vi "LIA Debugging FPGA.vi"() -> ()   [LabVIEW 2018]
uses:
  <vilib>/eio/EIONode/EIONode.xnode
  <vilib>/rvi/eio/common/nirviEmuTemplateMethod_errors.vi
  <vilib>/Platform/TimedLoop/XDataNode/wakeup.ctl
  <vilib>/Platform/TimedLoop/XDataNode/XDNodeRunTimeDep.lvlib
  <vilib>/Platform/TimedLoop/XDataNode/nitl_modes.ctl
  <vilib>/Platform/TimedLoop/XDataNode/timing_clust.ctl
  <vilib>/Platform/TimedLoop/XDataNode/XDataNode.xnode
  <instrlib>/_niInstr/Basic Elements/v1/FPGA/niInstr Basic Elements v1 FPGA.lvlib
  <instrlib>/_niInstr/DSP/v1/Shared/Public/IQ Data.ctl
  <instrlib>/_niInstr/DSP/v1/Shared/niInstr DSP v1 Shared.lvlib
  <instrlib>/_niInstr/DSP/v1/FPGA/niInstr DSP v1 FPGA.lvlib
  <instrlib>/_niInstr/DSP/v1/Xnodes/Public/Frequency Shift/niInstr DSP v1 Frequency Shift FPGA.xnode
  Shared/_NI PLL IP/FPGA/NI PLL IP FPGA.lvlib
  <vilib>/rvi/FXPMathLib/FxpMul/XNode/nifxpmath_Multiplier.xnode
  <vilib>/rvi/FXPMathLib/FxpAdd/XNode/nifxpmath_Add.xnode
  <instrlib>/_niInstr/DSP/v1/FPGA/Public/Sub VIs/Frequency Shift/Frequency Shift - 2 spc.vi
  Shared/lib/fpga/Lock-In Amplifier Example FPGA.lvlib
  <instrlib>/_niInstr/Streaming/v1/Common/Stream State.ctl
  <instrlib>/_niInstr/Streaming/v1/Common/niInstr Streaming v1 Common.lvlib
  <vilib>/rvi/FXPMathLib/sim/FxpSim.dll
  <instrlib>/_niInstr/DSP/v1/FPGA/Public/Sub VIs/Fractional Decimator/Fractional Decimator - 10 cps - 1x oc.vi
  <instrlib>/_niInstr/DSP/v1/FPGA/Public/Sub VIs/Fractional Decimator/Fractional Decimator - 1 spc - 2x oc.vi
  <userlib>/_NI Noise Generation IP/FPGA/Public/Low Level/AWGN FXP23x2.vi
  <instrlib>/_niInstr/Data Trigger/v1/Shared/Public/Edge Configuration Trigger Slope.ctl
  <instrlib>/_niInstr/Data Trigger/v1/Shared/niInstr Data Trigger v1 Shared.lvlib
  <instrlib>/_niInstr/Data Trigger/v1/Shared/Public/Edge Configuration FXP(+-,18,1).ctl
  Shared/SOS/Controls/IIR_Coeffs.ctl
  LIA Decimator1 Enum.ctl
  LIA Decimator0 Enum.ctl
panel:
  out "stream.overflow? 0":bool
  in  "stream.clear overflow 0":bool
  in  "lock-in.iir enable0 0":bool
  in  "lock-in.iir enable1 0":bool
  in  "lock-in.iir config1 0":T1={"b0"=0.015777587890625, "b1"=-0.030517578125, "-a1"=1.9578399658203125, "-a2"=-0.9589080810546875}
  in  "lock-in.iir decimation1 0":fxp<+,4,4> format="%#_3g"
  in  "lock-in.iir decimation0 0":fxp<+,4,4> format="%#_3g"
  in  "lock-in.iir config0 0":T1={"b0"=0.015777587890625, "b1"=-0.030517578125, "-a1"=1.9578399658203125, "-a2"=-0.9589080810546875}
  in  "lock-in.decimator1 0":T2
  in  "lock-in.fir1 fs 0":fxp<+,48,1>
  in  "nco.enable 0":bool=TRUE
  in  "nco.reset 0":bool
  in  "nco.frequency 0":fxp<+/-,48,0>
  in  "lock-in.fir0 fs 0":fxp<+,48,1>
  in  "lock-in.decimator0 0":T3
  in  "dpll.reset 1":bool
  in  "dpll.enable 1":bool
  in  "dpll.q 1":fxp<+/-,48,0>
  in  "dpll.m 1":i8
  in  "dpll.config 1":T4
  out "dpll.vco output 1":fxp<+/-,48,0>
  in  "dpll.channel 1":i32
  in  "dpll.channel 0":i32
  out "dpll.vco output 0":fxp<+/-,48,0>
  in  "dpll.config 0":T4
  in  "dpll.m 0":i8
  in  "dpll.q 0":fxp<+/-,48,0>
  in  "dpll.enable 0":bool
  in  "dpll.reset 0":bool
  in  "lock-in.enable 3":bool
  in  "lock-in.enable 2":bool
  in  "lock-in.enable 1":bool
  in  "lock-in.carrier 3":fxp<+/-,48,0>
  in  "lock-in.carrier 2":fxp<+/-,48,0>
  in  "lock-in.enable 0":bool
  in  "lock-in.channel select 3":i32
  in  "lock-in.carrier select 3":i32
  in  "lock-in.cic config valid 3":bool
  in  "lock-in.cic config 3":cluster{"factor":fxp<+,16,16>, "shift":i16}
  in  "lock-in.reset 3":bool
  out "stream.state 3":T6 caption="stream.state 0"
  out "stream.samples transferred 3":u64 caption="stream.samples transferred 0"
  out "stream.metadata 3":u64 caption="stream.metadata 0"
  in  "stream.num samples 3":u64 caption="stream.num samples 0"
  in  "stream.request state 3":T6 caption="stream.request state 0"
  in  "lock-in.channel select 2":i32
  in  "lock-in.carrier select 2":i32
  in  "lock-in.cic config valid 2":bool
  in  "lock-in.cic config 2":cluster{"factor":fxp<+,16,16>, "shift":i16}
  in  "lock-in.reset 2":bool
  out "stream.state 2":T6 caption="stream.state 0"
  out "stream.samples transferred 2":u64 caption="stream.samples transferred 0"
  out "stream.metadata 2":u64 caption="stream.metadata 0"
  in  "stream.num samples 2":u64 caption="stream.num samples 0"
  in  "stream.request state 2":T6 caption="stream.request state 0"
  out "pll.vco output 0":fxp<+/-,48,0>
  out "pll.vco output 1":fxp<+/-,48,0>
  out "stream.metadata 4":u64 caption="stream.metadata 0"
  out "stream.samples transferred 4":u64 caption="stream.samples transferred 0"
  out "stream.state 4":T6 caption="stream.state 0"
  in  "stream.request state 4":T6 caption="stream.request state 0"
  in  "stream.num samples 4":u64 caption="stream.num samples 0"
  in  "preview.channel select":i32
  in  "ao.reset 3":bool
  in  "ao.carrier 2":fxp<+/-,48,0>=0.010000000000001563
  in  "ao.level 2":fxp<+/-,18,1>
  in  "ao.reset 2":bool
  in  "ao.carrier 1":fxp<+/-,48,0>=0.010000000000001563
  in  "ao.level 1":fxp<+/-,18,1>
  in  "ao.reset 1":bool
  in  "ao.reset 0":bool
  in  "ao.carrier 0":fxp<+/-,48,0>=0.010000000000001563
  in  "ao.level 0":fxp<+/-,18,1>
  in  "lock-in.channel select 1":i32
  in  "lock-in.channel select 0":i32
  in  "stream.request state 1":T6 caption="stream.request state 0"
  in  "stream.num samples 1":u64 caption="stream.num samples 0"
  out "stream.metadata 1":u64 caption="stream.metadata 0"
  out "stream.samples transferred 1":u64 caption="stream.samples transferred 0"
  out "stream.state 1":T6 caption="stream.state 0"
  in  "lock-in.reset 1":bool
  in  "lock-in.cic config 1":cluster{"factor":fxp<+,16,16>, "shift":i16}
  in  "lock-in.cic config valid 1":bool
  in  "lock-in.carrier select 1":i32
  in  "lock-in.carrier select 0":i32
  in  "lock-in.cic config valid 0":bool
  in  "lock-in.cic config 0":cluster{"factor":fxp<+,16,16>, "shift":i16}
  in  "lock-in.reset 0":bool
  in  "lock-in.carrier 1":fxp<+/-,48,0>
  in  "lock-in.carrier 0":fxp<+/-,48,0>
  in  "ao.level 3":fxp<+/-,18,1>
  in  "pll.channel 1":i32
  in  "pll.reset 1":bool
  in  "pll.enable 1":bool
  in  "pll.config 1":T7={"quiescent frequency"=0.10000000000000142, "compensation"=0.0, "psd gain"=-18, "loop filter"={"order"=4, "cutoff"=6}}
  in  "pll.channel 0":i32
  in  "ao.noise gain 3":fxp<+,18,1>=0.01000213623046875
  in  "ao.carrier 3":fxp<+/-,48,0>=0.010000000000001563
  in  "ao.noise seeds 3":fxp<+,23,23>[](array[numeric])=[1.0, 12323.0]
  in  "pll.reset 0":bool
  in  "pll.enable 0":bool
  in  "stream.request state 0":T6
  in  "stream.num samples 0":u64
  out "stream.metadata 0":u64
  out "stream.samples transferred 0":u64
  out "stream.state 0":T6
  in  "pll.config 0":T7={"quiescent frequency"=0.10000000000000142, "compensation"=0.0, "psd gain"=-18, "loop filter"={"order"=4, "cutoff"=6}}
  out "IO Module\\InitDone":bool
  out "IO Module\\User Error":u32
  in  "IO Module\\User Command":u32
  in  "IO Module\\User Command Valid":bool
  out "IO Module\\User Command Ready":bool
  in  "IO Module\\User Command Arg 0":u32
  in  "IO Module\\User Command Arg 1":u32
  out "IO Module\\User Command Error":u16
  out "IO Module\\User Command Return":u32
  out "IO Module\\User Command Return Valid":bool
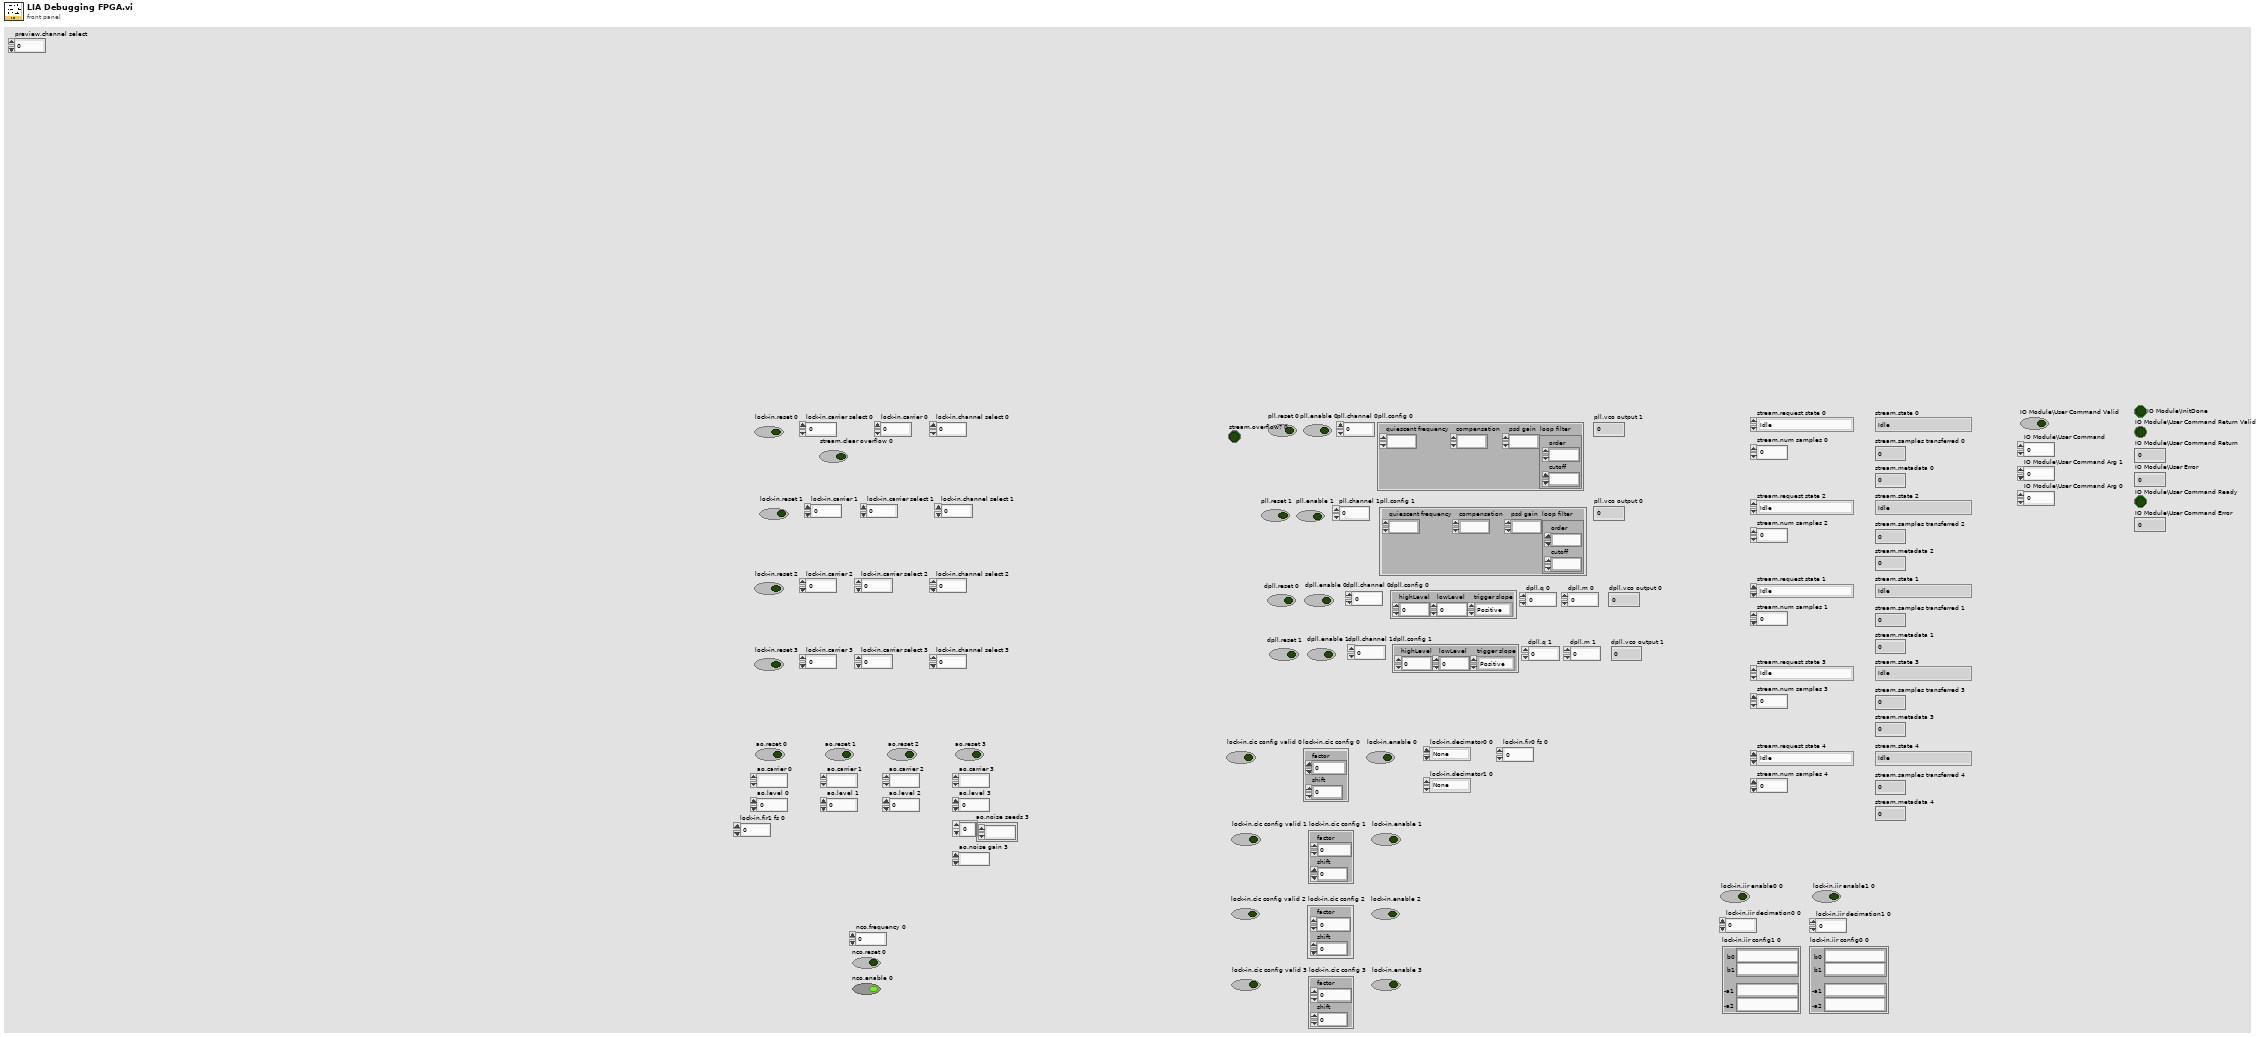
[diagram p1: front panel]
types:
  T1 = typedef "IIR_Coeffs.ctl" = cluster{"b0":fxp<+/-,18,2>, "b1":fxp<+/-,18,2>, "-a1":fxp<+/-,18,2>, "-a2":fxp<+/-,18,2>}
  T2 = typedef "LIA Decimator1 Enum.ctl" = enum16{"None", "FIR", "SOS"}
  T3 = typedef "LIA Decimator0 Enum.ctl" = enum16{"None", "CIC", "FIR", "4HB", "SOS", "4SOS"}
  T4 = typedef "niInstr Data Trigger v1 Shared.lvlib/Edge Configuration FXP(+-,18,1).ctl" = cluster{"highLevel":fxp<+/-,18,1>, "lowLevel":fxp<+/-,18,1>, "trigger slope":T5}
  T5 = typedef "niInstr Data Trigger v1 Shared.lvlib/Edge Configuration Trigger Slope.ctl" = enum8{"Positive", "Negative"}
  T6 = typedef "niInstr Streaming v1 Common.lvlib/Stream State.ctl" = enum8{"Idle", "Finite Transfer", "Continuous", "Done", "Error", "Not Ready", "Cancel"}
  T7 = cluster{"quiescent frequency":fxp<+/-,48,0>, "compensation":fxp<+/-,18,3>, "psd gain":i16, "loop filter":cluster{"order":i32, "cutoff":i8}}
  T8 = typedef "XDNodeRunTimeDep.lvlib/timing_clust.ctl" = cluster{"Expected End [f-1]":u64, "Actual End [f-1]":u64, "Finished Late? [f-1]":bool, "Expected End [i-1]":u64, "Actual End [i-1]":u64, "Finished Late? [i-1]":bool, "Expected Start [i]":u64, "Actual Start [i]":u64, "Expected Start [f]":u64, "Actual Start [f]":u64, "Source Name":string, "Structure Name":string, "Period":i64, "Deadline":i64, "Offset":i64, "Start":i64, "Priority":i32, "Timeout":i32, "Mode":T9, "Wakeup Reason":T10, "Error":errorcluster, "Source Type":string, "Secondary Source Type":string, "Global End Time":u64, "Global Start Time":u64, "Frame Duration":u64, "Iteration Duration":u64, "Assigned CPU":i32, "I/O Scan Engine Mode":u32}
  T9 = typedef "XDNodeRunTimeDep.lvlib/nitl_modes.ctl" = enum32{"No Change", "Process missed periods, maintain original phase", "Discard missed periods, maintain original phase", "Process missed periods, ignore original phase", "Discard missed periods, ignore original phase"}
  T10 = typedef "XDNodeRunTimeDep.lvlib/wakeup.ctl" = enum32{"Normal", "Aborted", "Asynchronous wakeup", "Timing source error", "Timed loop error", "Timeout"}
  T11 = cluster{"stream.num samples 0":u64, "stream.request state 0":T6, "stream.index 0":i16}
  T12 = typedef "niInstr DSP v1 Shared.lvlib/IQ Data.ctl" = cluster{"I":fxp<+/-,18,1>, "Q":fxp<+/-,18,1>, "overflow":bool}
  T13 = cluster{"stream.metadata 0":u64, "stream.samples transferred 0":u64, "stream.state 0":T6}
  T14 = typedef "niInstr DSP v1 Shared.lvlib/IQ Data - 25 bit.ctl" = cluster{"I":fxp<+/-,25,1>, "Q":fxp<+/-,25,1>, "overflow":bool}
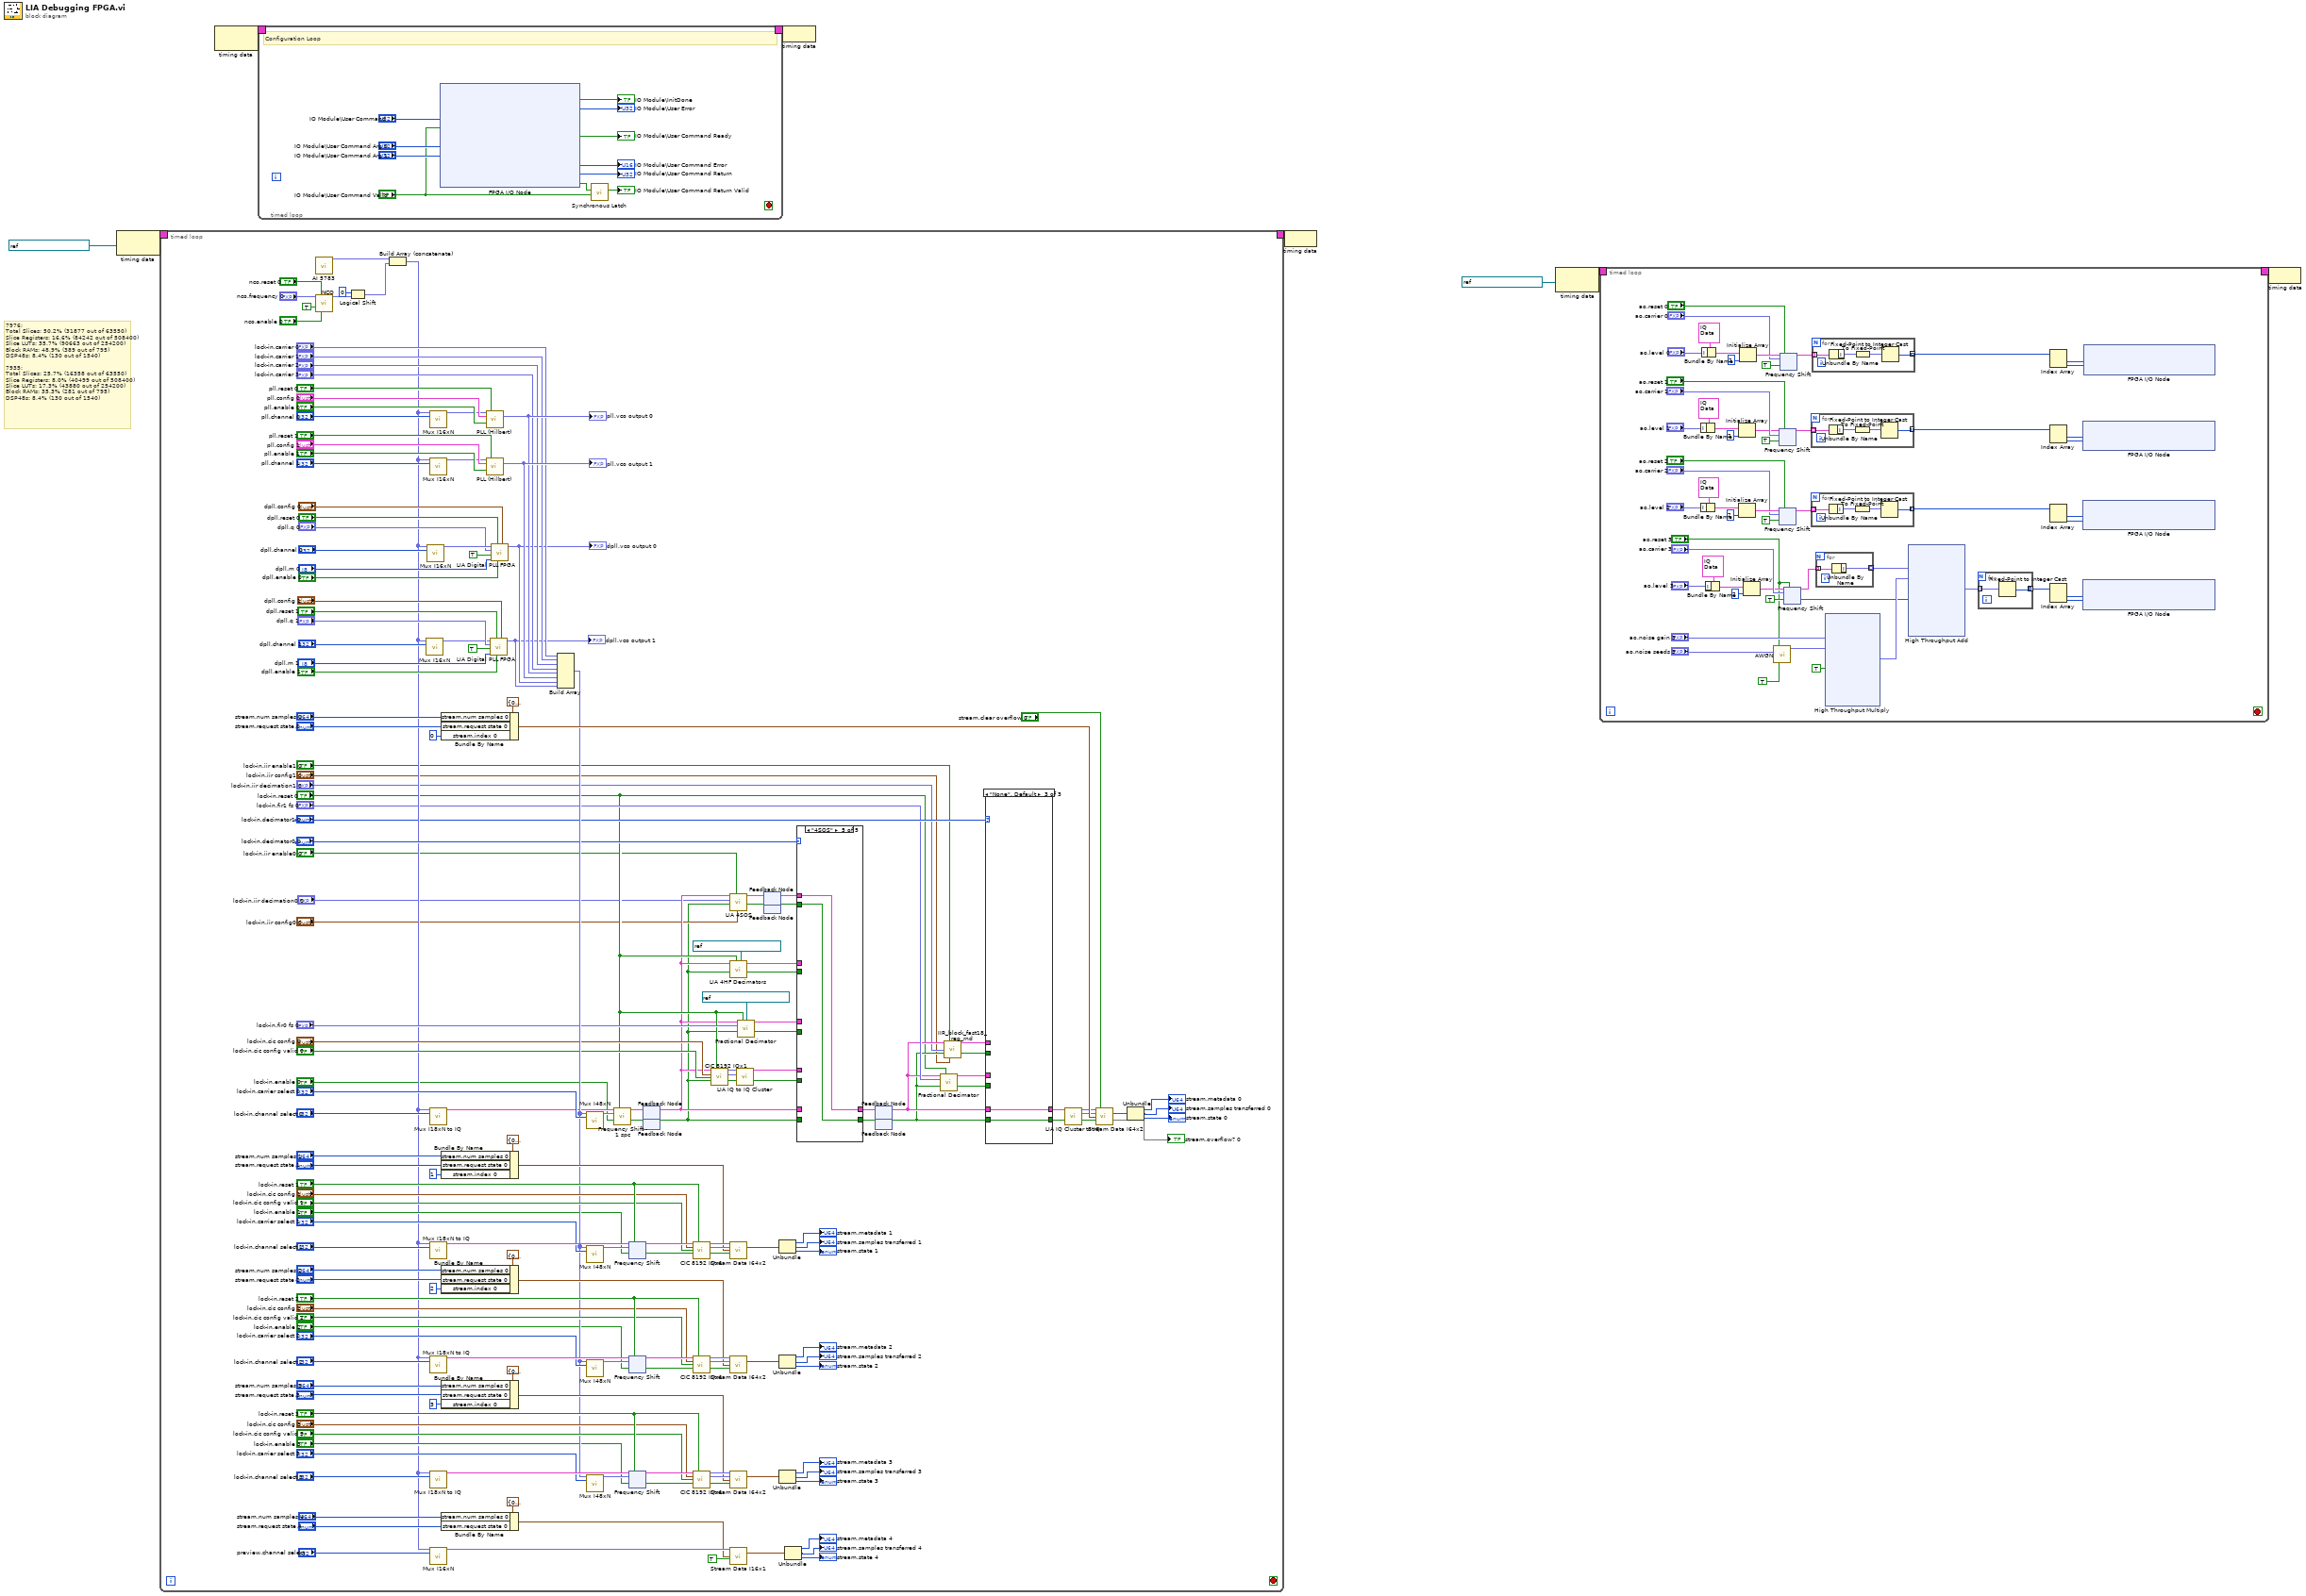
[diagram p0: block diagram]
diagram:
  # "7976:\nTotal Slices: 50.2% (31877 out of 63550)\nSlice Registers: 16.6% (84242 out of 508400)\nSlice LUTs: 35.7% (90663 out of 254200)\nBlock RAMs: 48.9% (389 out of 795)\nDSP48s: 8.4% (130 out of 1540)\n\n7935:\nTotal Slices: 25.7% (16358 out of 63550)\nSlice Registers: 8.0% (40499 out of 508400)\nSlice LUTs: 17.3% (43880 out of 254200)\nBlock RAMs: 35.3% (281 out of 795)\nDSP48s: 8.4% (130 out of 1540)"
  n1 = node-c288(refnum<k21> "IO Module\\Data Clock" ("Source Name")) -> (w8:T8)
  n2 = timed-loop {
    timing: w8 -> [_]
    timing-out: [_] -> w7
    stop <- _ stop-if-true
    n3 = call "AI 5783.vi"() -> ("i18x1"=w66:fxp<+/-,18,1>[])  [unwired: 14 in, 1 out]
    n4 = call <instrlib>:"NCO.vi"("frequency"="nco.frequency 0", "reset"="nco.reset 0", "input valid"=TRUE, "enable (T)"="nco.enable 0") -> ("cosine out"=w39:fxp<+/-,18,1>)  [unwired: 9 in, 2 out]
    n5 = Logical Shift(y=i16 0, x=w39) -> (x << y=w40:fxp<+/-,18,1>)
    n6 = Build Array (concatenate)(w66, w40) -> (w59:fxp<+/-,18,1>[])
    n7 = call "Mux I16xN.vi"("i16xn in"=w59, "index"="dpll.channel 1") -> ("i16 out"=w69:fxp<+/-,18,1>)  [unwired: 12 in, 1 out]
    n8 = call "Mux I16xN.vi"("i16xn in"=w59, "index"="dpll.channel 0") -> ("i16 out"=w81:fxp<+/-,18,1>)  [unwired: 12 in, 1 out]
    n9 = call "Mux I16xN.vi"("i16xn in"=w59, "index"="pll.channel 0") -> ("i16 out"=w185:fxp<+/-,18,1>)  [unwired: 12 in, 1 out]
    n10 = call "Mux I16xN.vi"("i16xn in"=w59, "index"="pll.channel 1") -> ("i16 out"=w179:fxp<+/-,18,1>)  [unwired: 12 in, 1 out]
    n11 = call "Mux I18xN to IQ.vi"("i16xn in"=w59, "index"="lock-in.channel select 0") -> ("output"=w28:T12)  [unwired: 12 in, 1 out]
    n12 = call "Mux I18xN to IQ.vi"("i16xn in"=w59, "index"="lock-in.channel select 1") -> ("output"=w167:T12)  [unwired: 12 in, 1 out]
    n13 = call "Mux I18xN to IQ.vi"("i16xn in"=w59, "index"="lock-in.channel select 2") -> ("output"=w133:T12)  [unwired: 12 in, 1 out]
    n14 = call "Mux I18xN to IQ.vi"("i16xn in"=w59, "index"="lock-in.channel select 3") -> ("output"=w112:T12)  [unwired: 12 in, 1 out]
    n15 = call "Mux I16xN.vi"("i16xn in"=w59, "index"="preview.channel select") -> ("i16 out"=w141:fxp<+/-,18,1>)  [unwired: 12 in, 1 out]
    n16 = Bundle By Name(cluster=T11 {"stream.num samples 0"=0, "stream.request state 0"=enum."Idle", "stream.index 0"=0} ("config"), "stream.num samples 0"="stream.num samples 0", "stream.request state 0"="stream.request state 0", "stream.index 0"=i16 0) -> (w170:T11)
    n17 = Bundle By Name(cluster=T11 {"stream.num samples 0"=0, "stream.request state 0"=enum."Idle", "stream.index 0"=0} ("config"), "stream.num samples 0"="stream.num samples 1", "stream.request state 0"="stream.request state 1", "stream.index 0"=i16 1) -> (w149:T11)
    n18 = Bundle By Name(cluster=T11 {"stream.num samples 0"=0, "stream.request state 0"=enum."Idle", "stream.index 0"=0} ("config"), "stream.num samples 0"="stream.num samples 2", "stream.request state 0"="stream.request state 2", "stream.index 0"=i16 2) -> (w115:T11)
    n19 = Bundle By Name(cluster=T11 {"stream.num samples 0"=0, "stream.request state 0"=enum."Idle", "stream.index 0"=0} ("config"), "stream.num samples 0"="stream.num samples 3", "stream.request state 0"="stream.request state 3", "stream.index 0"=i16 3) -> (w94:T11)
    n20 = Bundle By Name(cluster=T11 {"stream.num samples 0"=0, "stream.request state 0"=enum."Idle", "stream.index 0"=0} ("config"), "stream.num samples 0"="stream.num samples 4", "stream.request state 0"="stream.request state 4") -> (w137:T11)
    n21 = call "PLL (Hilbert).vi"("input"=w185, "reset"="pll.reset 0", "config"="pll.config 0", "enable"="pll.enable 0") -> ("output"=w134:fxp<+/-,48,0>)  [unwired: 11 in]
    "pll.vco output 0" <- w134
    n22 = call "PLL (Hilbert).vi"("input"=w179, "reset"="pll.reset 1", "config"="pll.config 1", "enable"="pll.enable 1") -> ("output"=w135:fxp<+/-,48,0>)  [unwired: 11 in]
    "pll.vco output 1" <- w135
    n23 = call "LIA Digital PLL FPGA.vi"("configuration"="dpll.config 1", "arm"="dpll.enable 1", "reset"="dpll.reset 1", "m"="dpll.m 1", "input valid"=TRUE, "q"="dpll.q 1", "I"=w69) -> ("frequency shift"=w65:fxp<+/-,48,0>)  [unwired: 1 in, 3 out]
    "dpll.vco output 1" <- w65
    n24 = call "LIA Digital PLL FPGA.vi"("configuration"="dpll.config 0", "arm"="dpll.enable 0", "reset"="dpll.reset 0", "m"="dpll.m 0", "input valid"=TRUE, "q"="dpll.q 0", "I"=w81) -> ("frequency shift"=w76:fxp<+/-,48,0>)  [unwired: 1 in, 3 out]
    "dpll.vco output 0" <- w76
    n25 = Build Array("lock-in.carrier 0", "lock-in.carrier 1", "lock-in.carrier 2", "lock-in.carrier 3", w134, w135, w76, w65) -> (w91:fxp<+/-,48,0>[])
    n26 = call "Mux I48xN.vi"("i48xn in"=w91, "index"="lock-in.carrier select 0") -> ("i48 out"=w25:fxp<+/-,48,0>)  [unwired: 13 in]
    n27 = call "Mux I48xN.vi"("i48xn in"=w91, "index"="lock-in.carrier select 1") -> ("i48 out"=w166:fxp<+/-,48,0>)  [unwired: 13 in]
    n28 = call "Mux I48xN.vi"("i48xn in"=w91, "index"="lock-in.carrier select 2") -> ("i48 out"=w132:fxp<+/-,48,0>)  [unwired: 13 in]
    n29 = call "Mux I48xN.vi"("i48xn in"=w91, "index"="lock-in.carrier select 3") -> ("i48 out"=w111:fxp<+/-,48,0>)  [unwired: 13 in]
    n30 = call <instrlib>:"Frequency Shift - 1 spc.vi"("data in"=w28, "reset"="lock-in.reset 0", "frequency shift"=w25, "input valid"="lock-in.enable 0") -> ("data out"=w27:T12, "output valid"=w26:bool)  [unwired: 8 in, 2 out]
    n31 = xnode "Frequency Shift"("data in"=w167, "reset"="lock-in.reset 1", "frequency shift"=w166, "input valid"="lock-in.enable 1") -> ("data out"=w165:T12, "output valid"=w164:bool)  [unwired: 2 in, 1 out]
    n32 = xnode "Frequency Shift"("data in"=w133, "reset"="lock-in.reset 2", "frequency shift"=w132, "input valid"="lock-in.enable 2") -> ("data out"=w131:T12, "output valid"=w130:bool)  [unwired: 2 in, 1 out]
    n33 = xnode "Frequency Shift"("data in"=w112, "reset"="lock-in.reset 3", "frequency shift"=w111, "input valid"="lock-in.enable 3") -> ("data out"=w110:T12, "output valid"=w109:bool)  [unwired: 2 in, 1 out]
    n34 = feedback-in #1(w27) -> ()
    n35 = feedback #1() -> (w17:T12)  [unwired: 1 in]
    n36 = feedback-in #2(w26) -> ()
    n37 = feedback #2() -> (w12:bool)  [unwired: 1 in]
    n38 = call "CIC 8192 IQx1.vi"("data"=w165, "reset"="lock-in.reset 1", "config"="lock-in.cic config 1", "config valid"="lock-in.cic config valid 1", "input valid"=w164) -> ("i out"=w160:fxp<+/-,64,1>, "q out"=w159:fxp<+/-,64,1>, "output valid"=w158:bool)  [unwired: 8 in]
    n39 = call "CIC 8192 IQx1.vi"("data"=w131, "reset"="lock-in.reset 2", "config"="lock-in.cic config 2", "config valid"="lock-in.cic config valid 2", "input valid"=w130) -> ("i out"=w126:fxp<+/-,64,1>, "q out"=w125:fxp<+/-,64,1>, "output valid"=w124:bool)  [unwired: 8 in]
    n40 = call "CIC 8192 IQx1.vi"("data"=w110, "reset"="lock-in.reset 3", "config"="lock-in.cic config 3", "config valid"="lock-in.cic config valid 3", "input valid"=w109) -> ("i out"=w105:fxp<+/-,64,1>, "q out"=w104:fxp<+/-,64,1>, "output valid"=w103:bool)  [unwired: 8 in]
    n41 = call "CIC 8192 IQx1.vi"("data"=w17, "reset"="lock-in.reset 0", "config"="lock-in.cic config 0", "config valid"="lock-in.cic config valid 0", "input valid"=w12) -> ("i out"=w46:fxp<+/-,64,1>, "q out"=w45:fxp<+/-,64,1>, "output valid"=w61:bool)  [unwired: 8 in]
    n42 = call "LIA 4HF Decimators.vi"("clock x 2"=refnum<k21> "IO Module\\Data Clock 2x", "reset"="lock-in.reset 0", "input valid"=w12, "data in"=w17) -> ("output valid"=w50:bool, "data out"=w51:T12)  [unwired: 6 in]
    n43 = call "LIA 4SOS.vi"("lock-in.iir config0 0"="lock-in.iir config0 0", "lock-in.iir enable0 0"="lock-in.iir enable0 0", "input valid"=w12, "lock-in.iir decimation0 0"="lock-in.iir decimation0 0", "IQ_Data_In"=w17) -> ("output valid"=w14:bool, "IQ_Data_Out"=w15:T12)  [unwired: 5 in]
    n44 = call "Stream Data I64x2.vi"("i in"=w160, "q in"=w159, "config"=w149, "input valid"=w158) -> ("status"=w157:T13)  [unwired: 11 in]
    n45 = call "Stream Data I64x2.vi"("i in"=w126, "q in"=w125, "config"=w115, "input valid"=w124) -> ("status"=w123:T13)  [unwired: 11 in]
    n46 = call "Stream Data I64x2.vi"("i in"=w105, "q in"=w104, "config"=w94, "input valid"=w103) -> ("status"=w102:T13)  [unwired: 11 in]
    n47 = call "Stream Data I16x1.vi"("i in"=w141, "config"=w137, "input valid"=TRUE) -> ("status"=w143:T13)  [unwired: 12 in]
    n48 = call "LIA IQ to IQ Cluster.vi"("i in"=w46, "q in"=w45) -> ("data out"=w44:T12)  [unwired: 13 in]
    n49 = call-poly <instrlib>:"Fractional Decimator.vi"("data in"=w17, "reset"="lock-in.reset 0", "clock x 2"=refnum<k21> "IO Module\\Data Clock 2x", "output sample rate"="lock-in.fir0 fs 0", "input valid"=w12) -> ("data out"=w53:T12, "output valid"=w54:bool)  [unwired: 8 in, 1 out]
    n50 = feedback-in #3(w15) -> ()
    n51 = feedback #3() -> (w10:T12)  [unwired: 1 in]
    n52 = feedback-in #4(w14) -> ()
    n53 = feedback #4() -> (w9:bool)  [unwired: 1 in]
    n54 = Unbundle(w157) -> ("stream.metadata 0"=→"stream.metadata 1":u64, "stream.samples transferred 0"=→"stream.samples transferred 1":u64, "stream.state 0"=→"stream.state 1":T6)
    n55 = Unbundle(w123) -> ("stream.metadata 0"=→"stream.metadata 2":u64, "stream.samples transferred 0"=→"stream.samples transferred 2":u64, "stream.state 0"=→"stream.state 2":T6)
    n56 = Unbundle(w102) -> ("stream.metadata 0"=→"stream.metadata 3":u64, "stream.samples transferred 0"=→"stream.samples transferred 3":u64, "stream.state 0"=→"stream.state 3":T6)
    n57 = Unbundle(w143) -> ("stream.metadata 0"=→"stream.metadata 4":u64, "stream.samples transferred 0"=→"stream.samples transferred 4":u64, "stream.state 0"=→"stream.state 4":T6)
    n58 = case shown="\"4SOS\"" "lock-in.decimator0 0" {
      tunnel: [w196 w198 w200 w202 w203] -> w33
      tunnel: w61 -> [_ w198 _ _ _]
      tunnel: w54 -> [_ _ w200 _ _]
      tunnel: w12 -> [w196 _ _ _ _]
      tunnel: w53 -> [_ _ w199 _ _]
      tunnel: w17 -> [w195 _ _ _ _]
      tunnel: w51 -> [_ _ _ w201 _]
      tunnel: w50 -> [_ _ _ w202 _]
      tunnel: [w195 w197 w199 w201 w204] -> w35
      tunnel: w44 -> [_ w197 _ _ _]
      tunnel: w10 -> [_ _ _ _ w204]
      tunnel: w9 -> [_ _ _ _ w203]
      frame "None", Default {
      }
      frame "CIC" {
      }
      frame "FIR" {
      }
      frame "4HB" {
      }
      frame "4SOS" {
      }
    }
    n59 = feedback #5() -> (w34:T12)  [unwired: 1 in]
    n60 = feedback-in #5(w35) -> ()
    n61 = feedback #6() -> (w32:bool)  [unwired: 1 in]
    n62 = feedback-in #6(w33) -> ()
    n63 = call-poly <instrlib>:"Fractional Decimator.vi"("data in"=w34, "reset"="lock-in.reset 0", "output sample rate"="lock-in.fir1 fs 0", "input valid"=w32) -> ("data out"=w43:T14, "output valid"=w42:bool)  [unwired: 9 in, 1 out]
    n64 = call "IIR_block_fast18_reg_rnd.vi"("IQ_Data_In"=w34, "enable"="lock-in.iir enable1 0", "Decimation Factor (-1)"="lock-in.iir decimation1 0", "Valid In"=w32, "IIR 2 coeffs"="lock-in.iir config1 0") -> ("IQ_Data_Out"=w37:T12, "output valid"=w36:bool)  [unwired: 9 in]
    n65 = case shown="\"None\", Default" "lock-in.decimator1 0" {
      tunnel: [w189 w191 w194] -> w49
      tunnel: w32 -> [_ _ w194]
      tunnel: w34 -> [_ _ w193]
      tunnel: [w190 w192 w193] -> w22
      tunnel: w43 -> [w190 _ _]
      tunnel: w42 -> [w189 _ _]
      tunnel: w37 -> [_ w192 _]
      tunnel: w36 -> [_ w191 _]
      frame "FIR" {
      }
      frame "SOS" {
      }
      frame "None", Default {
      }
    }
    n66 = call "LIA IQ Cluster to IQ.vi"("data in"=w22) -> ("i in"=w21:fxp<+/-,64,1>, "q in"=w20:fxp<+/-,64,1>)  [unwired: 13 in]
    n67 = call "Stream Data I64x2.vi"("i in"=w21, 1:"stream.clear overflow 0", "q in"=w20, "config"=w170, "input valid"=w49) -> ("status"=w178:T13, 10:→"stream.overflow? 0")  [unwired: 9 in]
    n68 = Unbundle(w178) -> ("stream.metadata 0"=→"stream.metadata 0":u64, "stream.samples transferred 0"=→"stream.samples transferred 0":u64, "stream.state 0"=→"stream.state 0":T6)
  }
  n69 = node-c288() -> (w2:T8)  [unwired: 1 in]
  n70 = timed-loop {
    timing: w2 -> [_]
    timing-out: [_] -> w1
    stop <- _ stop-if-true
    # "Configuration Loop"
    n71 = xnode "FPGA I/O Node"("IO Module\\User Command"="IO Module\\User Command", "IO Module\\User Command Valid"="IO Module\\User Command Valid", "IO Module\\User Command Arg 0"="IO Module\\User Command Arg 0", "IO Module\\User Command Arg 1"="IO Module\\User Command Arg 1") -> ("IO Module\\InitDone"=→"IO Module\\InitDone":bool, "IO Module\\Clip Error Code"=→"IO Module\\User Error":u32, "IO Module\\User Command Ready"=→"IO Module\\User Command Ready":bool, "IO Module\\User Command Error"=→"IO Module\\User Command Error":u16, "IO Module\\User Command Return"=→"IO Module\\User Command Return":u32, "IO Module\\User Command Return Valid"=w235:bool)  [unwired: 10 in, 10 out]
    n72 = call <instrlib>:"Synchronous Latch.vi"("clear"="IO Module\\User Command Valid", "set"=w235) -> ("out"=→"IO Module\\User Command Return Valid":bool)  [unwired: 9 in]
  }
  n73 = node-c288(w1) -> ()
  n74 = node-c288(w7) -> ()
  n75 = node-c288(refnum<k21> "IO Module\\Data Clock" ("Source Name")) -> (w5:T8)
  n76 = timed-loop {
    timing: w5 -> [_]
    timing-out: [_] -> w4
    stop <- _ stop-if-true
    n77 = Bundle By Name(cluster=T12 {"I"=0.0, "Q"=0.0, "overflow"=FALSE} ("output"), "I"="ao.level 1") -> (w268:T12)
    n78 = Bundle By Name(cluster=T12 {"I"=0.0, "Q"=0.0, "overflow"=FALSE} ("output"), "I"="ao.level 2") -> (w258:T12)
    n79 = Bundle By Name(cluster=T12 {"I"=0.0, "Q"=0.0, "overflow"=FALSE} ("output"), "I"="ao.level 0") -> (w283:T12)
    n80 = Bundle By Name(cluster=T12 {"I"=0.0, "Q"=0.0, "overflow"=FALSE} ("output"), "I"="ao.level 3") -> (w292:T12)
    n81 = Initialize Array(w268, 2 ("dimension size")) -> (w264:T12[])
    n82 = Initialize Array(w258, 2 ("dimension size")) -> (w262:T12[])
    n83 = Initialize Array(w283, 2 ("dimension size")) -> (w287:T12[])
    n84 = Initialize Array(w292, 2 ("dimension size")) -> (w288:T12[])
    n85 = call-poly <userlib>:"AWGN.vi"("reset"="ao.reset 3", "seeds"="ao.noise seeds 3", "ready"=TRUE) -> ("output 0"=w295:fxp<+/-,23,4>[])  [unwired: 10 in, 2 out]
    n86 = xnode "Frequency Shift"("data in"=w264, "reset"="ao.reset 1", "frequency shift"="ao.carrier 1", "input valid"=TRUE) -> ("data out"=w272:T12[])  [unwired: 2 in, 2 out]
    n87 = xnode "Frequency Shift"("data in"=w262, "reset"="ao.reset 2", "frequency shift"="ao.carrier 2", "input valid"=TRUE) -> ("data out"=w254:T12[])  [unwired: 2 in, 2 out]
    n88 = xnode "Frequency Shift"("data in"=w287, "reset"="ao.reset 0", "frequency shift"="ao.carrier 0", "input valid"=TRUE) -> ("data out"=w279:T12[])  [unwired: 2 in, 2 out]
    n89 = xnode "Frequency Shift"("data in"=w288, "reset"="ao.reset 3", "frequency shift"="ao.carrier 3", "input valid"=TRUE) -> ("data out"=w303:T12[], "output valid"=w300:bool)  [unwired: 2 in, 1 out]
    n90 = for {
      tunnel: w272 -> [w319] mode=indexing
      tunnel: [w320] -> w273 mode=indexing
      n91 = Unbundle By Name(w319) -> ("I"=w318:fxp<+/-,18,1>)
      n92 = To Fixed-Point(number=w318) -> (fixed-point=w317:fxp<+/-,16,1>)  [unwired: 1 in]
      n93 = Fixed-Point to Integer Cast(1:w317) -> (0:w320:i16)
    }
    n94 = for {
      tunnel: w254 -> [w306] mode=indexing
      tunnel: [w307] -> w253 mode=indexing
      n95 = Unbundle By Name(w306) -> ("I"=w305:fxp<+/-,18,1>)
      n96 = To Fixed-Point(number=w305) -> (fixed-point=w304:fxp<+/-,16,1>)  [unwired: 1 in]
      n97 = Fixed-Point to Integer Cast(1:w304) -> (0:w307:i16)
    }
    n98 = for {
      tunnel: w279 -> [w332] mode=indexing
      tunnel: [w333] -> w278 mode=indexing
      n99 = Unbundle By Name(w332) -> ("I"=w331:fxp<+/-,18,1>)
      n100 = To Fixed-Point(number=w331) -> (fixed-point=w330:fxp<+/-,16,1>)  [unwired: 1 in]
      n101 = Fixed-Point to Integer Cast(1:w330) -> (0:w333:i16)
    }
    n102 = for {
      tunnel: w303 -> [w346] mode=indexing
      tunnel: [w345] -> w299 mode=indexing
      n103 = Unbundle By Name(w346) -> ("I"=w345:fxp<+/-,18,1>)
    }
    n104 = xnode ("High Throughput Multiply")("x"="ao.noise gain 3", "y"=w295, "input valid"=TRUE) -> ("x*y"=w302:fxp<+/-,41,5>[])  [unwired: 1 in, 2 out]
    n105 = xnode ("High Throughput Add")("x"=w299, "y"=w302, "input valid"=w300) -> ("x+y"=w294:fxp<+/-,16,1>[])  [unwired: 1 in, 2 out]
    n106 = for {
      tunnel: w294 -> [w344] mode=indexing
      tunnel: [w343] -> w263 mode=indexing
      n107 = Fixed-Point to Integer Cast(1:w344) -> (0:w343:i16)
    }
    n108 = Index Array(array=w278) -> (element #1=w277:i16, element #2=w276:i16)  [unwired: 2 in]
    n109 = Index Array(array=w273) -> (element #1=w274:i16, element #2=w275:i16)  [unwired: 2 in]
    n110 = Index Array(array=w253) -> (element #1=w252:i16, element #2=w251:i16)  [unwired: 2 in]
    n111 = Index Array(array=w263) -> (element #1=w250:i16, element #2=w249:i16)  [unwired: 2 in]
    n112 = xnode "FPGA I/O Node"("IO Module\\AO 1 Data N-1 Data Clock"=w274, "IO Module\\AO 1 Data N Data Clock"=w275) -> ()  [unwired: 2 in, 2 out]
    n113 = xnode "FPGA I/O Node"("IO Module\\AO 2 Data N-1 Data Clock"=w252, "IO Module\\AO 2 Data N Data Clock"=w251) -> ()  [unwired: 2 in, 2 out]
    n114 = xnode "FPGA I/O Node"("IO Module\\AO 3 Data N-1 Data Clock"=w250, "IO Module\\AO 3 Data N Data Clock"=w249) -> ()  [unwired: 2 in, 2 out]
    n115 = xnode "FPGA I/O Node"("IO Module\\AO 0 Data N-1 Data Clock"=w277, "IO Module\\AO 0 Data N Data Clock"=w276) -> ()  [unwired: 2 in, 2 out]
  }
  n116 = node-c288(w4) -> ()
